vi "Load Abort.vi"(8 "error in (no error)":errorcluster, 11 "DiscreteRangeControl in":refnum<class "DiscreteRangeControl.lvclass">) -> (0 "error out":errorcluster, 3 "DiscreteRangeControl out":refnum<class "DiscreteRangeControl.lvclass">)   [LabVIEW 2020, in "VolatusControl.lvlib" / "DiscreteRangeControl.lvclass"]
uses:
  DiscreteRangeControl.lvclass
  DiscreteRangeControl.lvclass/DiscreteRangeControl.ctl
  lv-cdm/CDM-Config/Config Element/Config Element.lvclass
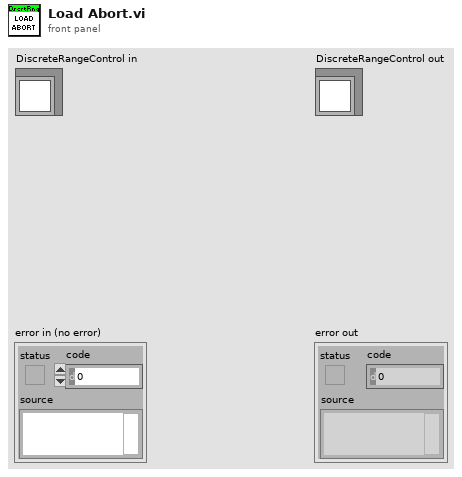
[diagram p1: front panel]
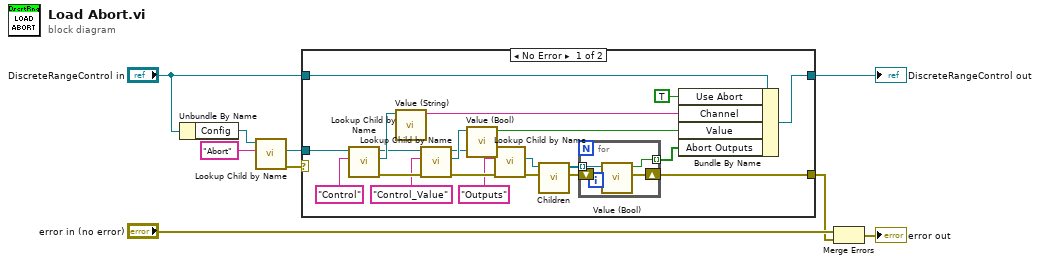
[diagram p0: block diagram]
diagram:
  n1 = Unbundle By Name("DiscreteRangeControl in") -> ("Config"=w8:refnum<class "Config Element.lvclass">)
  n2 = call "Lookup Child by Name.vi"("Name"="Abort", "Config Element in"=w8) -> ("error out"=w4:errorcluster, "Child"=w5:refnum<class "Config Element.lvclass">)  [unwired: 6 in, 2 out]
  n3 = case shown="No Error" w4 {
    tunnel: "DiscreteRangeControl in" -> [w16 w35]
    tunnel: w5 -> [w28 _]
    tunnel: [w12 w35] -> w3
    tunnel: [w11 _] -> w1
    frame No Error {
      n4 = call "Lookup Child by Name.vi"("Name"="Control", "Config Element in"=w28) -> ("error out"=w29:errorcluster, "Child"=w26:refnum<class "Config Element.lvclass">, "Config Element out"=w24:refnum<class "Config Element.lvclass">)  [unwired: 6 in, 1 out]
      n5 = call "Value (String).vi"("Config Element in"=w26) -> ("String Value"=w14:string)  [unwired: 9 in, 1 out]
      n6 = call "Lookup Child by Name.vi"("error in (no error)"=w29, "Name"="Control_Value", "Config Element in"=w24) -> ("error out"=w30:errorcluster, "Child"=w23:refnum<class "Config Element.lvclass">, "Config Element out"=w21:refnum<class "Config Element.lvclass">)  [unwired: 5 in, 1 out]
      n7 = call "Value (Bool).vi"("Config Element in"=w23) -> ("Bool Value"=w13:bool)  [unwired: 9 in, 1 out]
      n8 = call "Lookup Child by Name.vi"("error in (no error)"=w30, "Name"="Outputs", "Config Element in"=w21) -> ("error out"=w19:errorcluster, "Child"=w20:refnum<class "Config Element.lvclass">)  [unwired: 5 in, 2 out]
      n9 = call "Children.vi"("error in (no error)"=w19, "Config Element in"=w20) -> ("error out"=w18:errorcluster, "Elements"=w17:refnum<class "Config Element.lvclass">[])  [unwired: 8 in]
      n10 = for {
        shift-right: [w32] -> w11
        shift-left: w18 -> [w33]
        tunnel: w17 -> [w34] mode=indexing
        tunnel: [w31] -> w15 mode=indexing
        n11 = call "Value (Bool).vi"("error in (no error)"=w33, "Config Element in"=w34) -> ("error out"=w32:errorcluster, "Bool Value"=w31:bool)  [unwired: 8 in]
      }
      n12 = Bundle By Name(cluster=w16, "Use Abort"=TRUE, "Channel"=w14, "Value"=w13, "Abort Outputs"=w15) -> (w12:refnum<class "DiscreteRangeControl.lvclass">)
    }
    frame Error {
      # "Abort not configured"
    }
  }
  "DiscreteRangeControl out" <- w3
  n13 = Merge Errors("error in (no error)", w1) -> (→"error out":errorcluster)
